vi "Adjust Splitter.vi"(8 "error in":errorcluster, 10 "Show":bool, 11 "Bottom Panel in":refnum<class "BottomDock.lvclass">) -> (0 "error out":errorcluster, 3 "Bottom Panel out":refnum<class "BottomDock.lvclass">)   [LabVIEW 2023, in "Docking.lvlib" / "BottomDock.lvclass"]
doc: "This class is designed so that ancestor classes can rescale the UI to fit the actor core of the ancestor UI."
uses:
  BottomDock.lvclass
  C:/Users/Public/Documents/Development/builds/Framework/Engine.lvlibp/Engine/Library/Engine.lvclass
  C:/Users/Public/Documents/Development/Application/Docking/Panels/Docking/Docking.lvclass
  Docking/Docking.lvclass/Docking.ctl
  Docking/Read Splitter Refnum.vi
  Docking/Read InitialPosition.vi
  builds/Framework/Engine.lvlibp/Engine/Accessors/Read VI Ref.vi
  builds/Framework/Engine.lvlibp/Engine/Library/Engine.lvclass
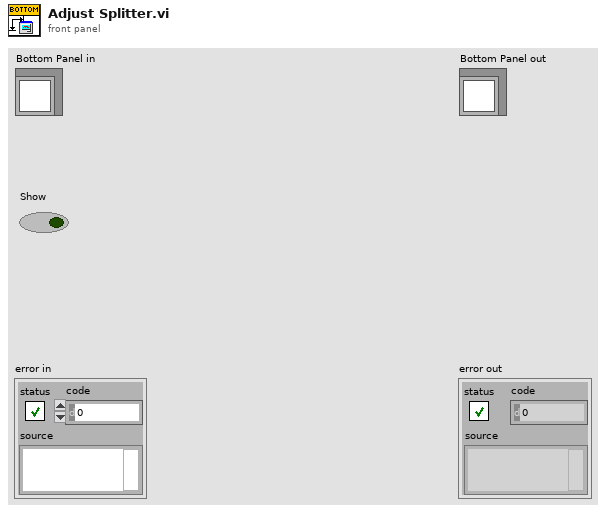
[diagram p1: front panel]
types:
  T1 = typedef "LVPointTypeDef.ctl" = cluster{"Horizontal":i16, "Vertical":i16}
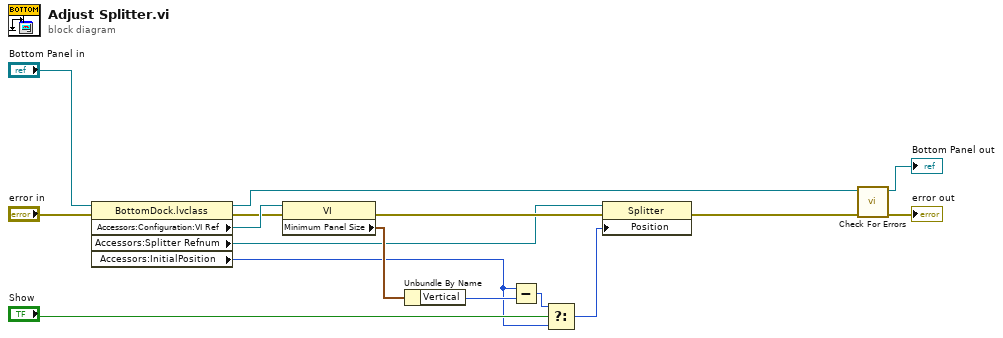
[diagram p0: block diagram]
diagram:
  n1 = property class="BottomDock.lvclass"(reference="Bottom Panel in", error in="error in") -> (reference out=w3:refnum<class "BottomDock.lvclass">, error out=w11:errorcluster, "Accessors:Configuration:VI Ref"=w12:refnum<vi>, "Accessors:Splitter Refnum"=w2:refnum<vi>, "Accessors:InitialPosition"=w1:i32)
  n2 = property class="VI"(reference=w12, error in=w11) -> (error out=w5:errorcluster, "Minimum Panel Size"=w10:T1)  [unwired: 1 out]
  n3 = Unbundle By Name(w10) -> ("Vertical"=w8:i16)
  n4 = Subtract(x=w1, y=w8) -> (x-y=w9:i32)
  n5 = Select(t=w9, s="Show", f=w1) -> (s? t:f=w6:i32)
  n6 = property class="Splitter"(reference=w2, error in=w5, "Position"=w6) -> (error out=w4:errorcluster)  [unwired: 1 out]
  n7 = call "Check For Errors.vi"("error in"=w4, "Engine in"=w3) -> ("error out"=→"error out":errorcluster, "Engine out"=→"Bottom Panel out":refnum<class "BottomDock.lvclass">)  [unwired: 8 in]
